vi "Teleop.vi"(0 "Call Context":T2, 5 "Match Info":T1={"Autonomous Elapsed Seconds"=0.0, "TeleOp Elapsed Seconds"=0.0, "Disabled Elapsed Seconds"=0.0, "Visited Autonomous"=FALSE, "Visited TeleOp"=FALSE, "Visited Disabled"=FALSE, "Autonomous Settings"={"Autonomous Style"=enum."Independent", "VI Refnum"=refnum}}) -> ()   [LabVIEW 2020]
doc: "This VI is called for each TeleOp packet received from the DS where the robot is not disabled. It is often used to read from the joysticks and update I/O or to update setpoints for timed control loops. It should complete and return within 20 milliseconds or it may miss DS packets."
uses:
  <vilib>/Rock Robotics/WPI/DriverStation/WPI_DriverStationDerivedRobotMode.ctl
  <vilib>/Rock Robotics/WPI/DriverStation/WPI_DriverStationMatch Info.ctl
  <vilib>/Rock Robotics/WPI/Utilities/WPI_GetSetVariantRefNum.vi
  <vilib>/Rock Robotics/Network Tables/NT Read Boolean.vi
  <vilib>/Rock Robotics/Network Tables/NT Read Number.vi
  LX.vi
panel:
  out "Sample Slider 0":dbl(slide) scale=0.0..5.0
  out "Sample Boolean 1":bool
  out "Sample Boolean 0":bool
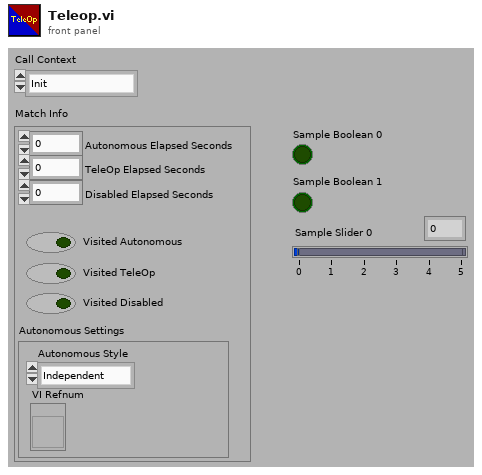
[diagram p1: front panel]
types:
  T1 = typedef "WPI_DriverStationMatch Info.ctl" = cluster{"Autonomous Elapsed Seconds":dbl, "TeleOp Elapsed Seconds":dbl, "Disabled Elapsed Seconds":dbl, "Visited Autonomous":bool, "Visited TeleOp":bool, "Visited Disabled":bool, "Autonomous Settings":cluster{"Autonomous Style":enum16{"Iterative", "Independent"}, "VI Refnum":refnum<vi>}}
  T2 = typedef "WPI_DriverStationDerivedRobotMode.ctl" = enum16{"Init", "Execute", "Stop"}
  T3 = typedef "WPI_JoystickDevRef.ctl" = cluster{"Device":T4}
  T4 = typedef "WPI_JoystickDeviceEnum.ctl" = enum16{"USB 0", "USB 1", "USB 2", "USB 3", "USB 4", "USB 5"}
  T5 = typedef "WPI_RobotDriveDevRef.ctl" = cluster{"DevStatus":errorcluster, "Motors[]":T6[], "Square Inputs":bool, "Max Output":dbl}
  T6 = typedef "WPI_MotorControlDeviceRef.ctl" = cluster{"DeviceStatus":errorcluster, "Type":T7, "PWM":cluster{"PWM Channel":T8, "DeadBand":T9}, "CAN":cluster{"Device Number":u8, "SetOutput VI Ref":variant, "GetOutput VI Ref":variant, "Enable VI Ref":variant, "Disable VI Ref":variant, "Data":variant}, "Invert":bool, "DIO PWM":cluster{"PWM \"Enable\" Channel":T8, "DIOChannel":T10, "PWM Rate":dbl}}
  T7 = typedef "WPI_MotorControlType.ctl" = enum16{"PWM", "CAN", "DIO PWM"}
  T8 = typedef "FPGA_DIOPWMChannel.ctl" = enum8{"PWM 0", "PWM 1", "PWM 2", "PWM 3", "PWM 4", "PWM 5", "PWM 6", "PWM 7", "PWM 8", "PWM 9", "PWM MXP 0", "PWM MXP 1", "PWM MXP 2", "PWM MXP 3", "PWM MXP 4", "PWM MXP 5", "PWM MXP 6", "PWM MXP 7", "PWM MXP 8", "PWM MXP 9", "Invalid"}
  T9 = typedef "WPI_PWMDeadband.ctl" = cluster{"Name":string, "maxPositivePwm":i32, "minPositivePwm":i32, "centerPwm":i32, "maxNegativePwm":i32, "minNegativePwm":i32, "angularRange":u16}
  T10 = typedef "FPGA_DIOChannel.ctl" = enum8{"DIO 0", "DIO 1", "DIO 2", "DIO 3", "DIO 4", "DIO 5", "DIO 6", "DIO 7", "DIO 8", "DIO 9", "DIO MXP 0", "DIO MXP 1", "DIO MXP 2", "DIO MXP 3", "DIO MXP 4", "DIO MXP 5", "DIO MXP 6", "DIO MXP 7", "DIO MXP 8", "DIO MXP 9", "DIO MXP 10", "DIO MXP 11", "DIO MXP 12", "DIO MXP 13", "DIO MXP 14", "DIO MXP 15", "SPI Port CS1", "SPI Port CS2", "SPI Port CS3", "SPI Port MISO", "SPI Port MOSI", "Invalid"}
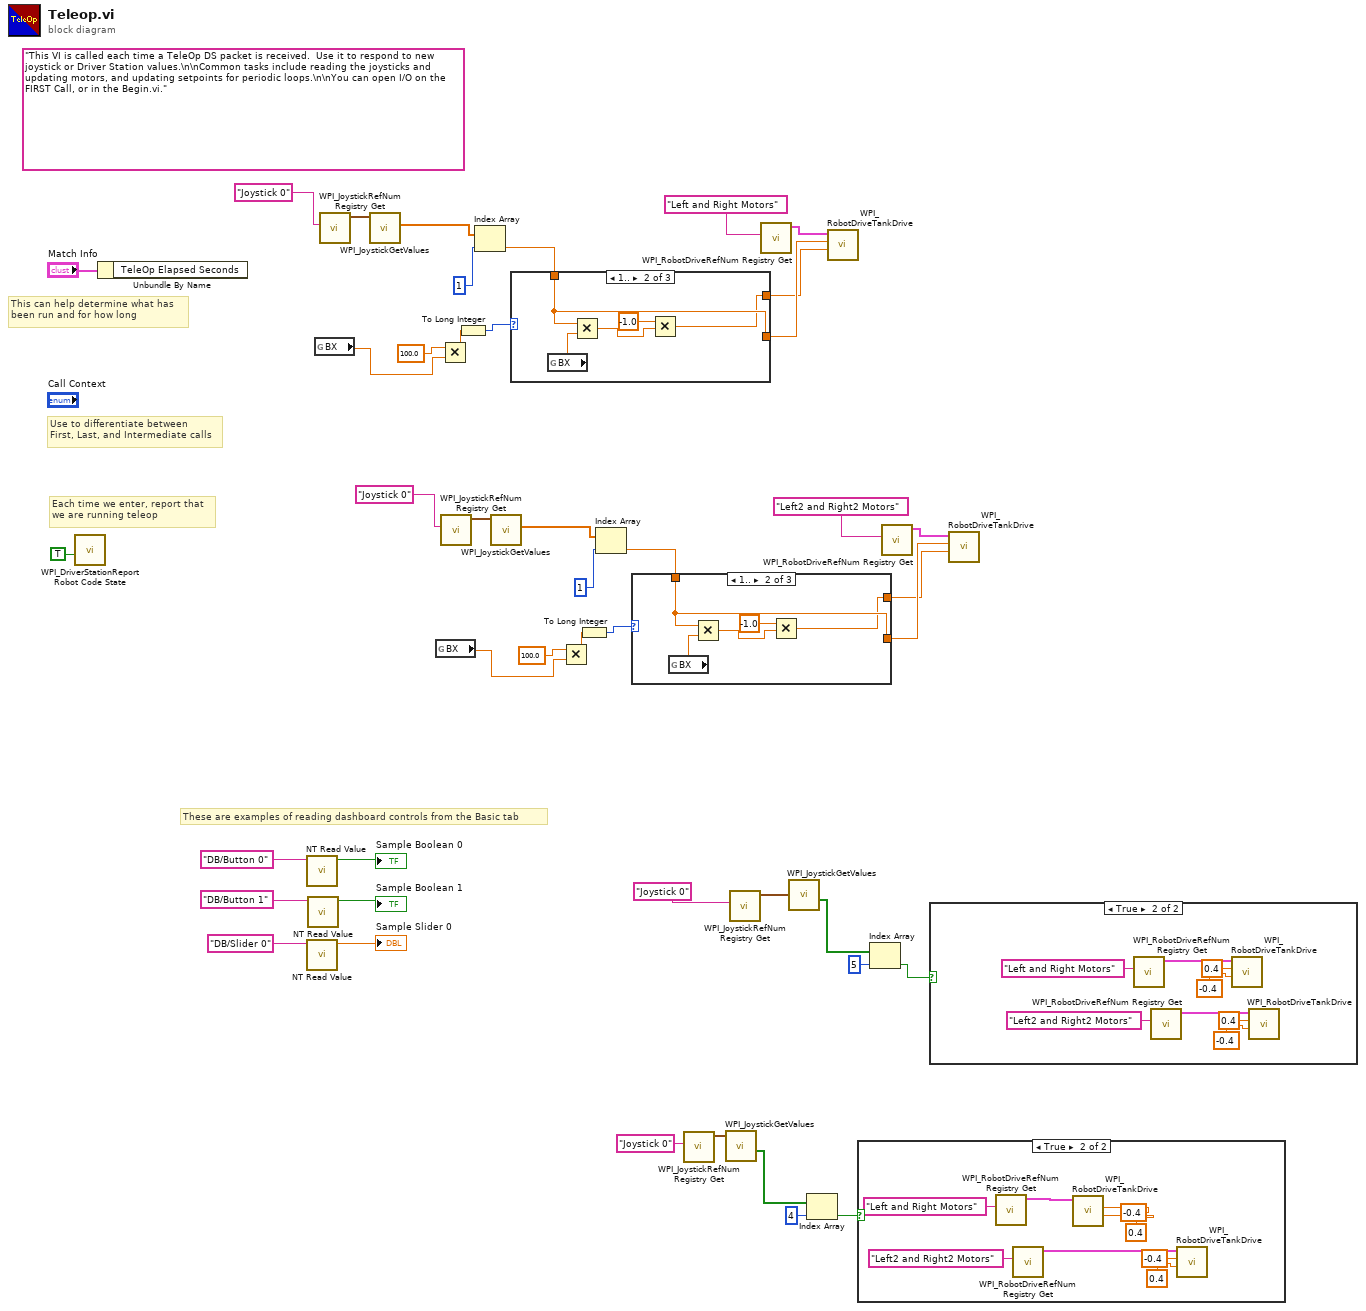
[diagram p0: block diagram]
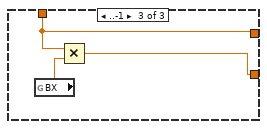
[diagram p3: hidden frame]
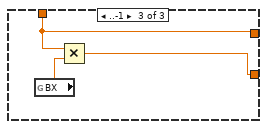
[diagram p5: hidden frame]
diagram:
  (unwired) "This VI is called each time a TeleOp DS packet is received.  Use it to respond to new joystick or Driver Station values.\n\nCommon tasks include reading the joysticks and updating motors, and updating setpoints for periodic loops.\n\nYou can open I/O on the FIRST Call, or in the Begin.vi."
  # "These are examples of reading dashboard controls from the Basic tab"
  # "Each time we enter, report that\nwe are running teleop"
  # "Use to differentiate between\nFirst, Last, and Intermediate calls"
  # "This can help determine what has\nbeen run and for how long"
  n1 = call <vilib>:"WPI_DriverStationReport Robot Code State.vi"("TeleOp"=TRUE ("Autonomous")) -> ()  [unwired: 10 in, 1 out]
  n2 = Unbundle By Name("Match Info") -> ()  [unwired: 1 out]
  n3 = call-poly <vilib>:"NT Read Value.vi"("Name"="DB/Button 0" ("refnum name")) -> ("Boolean"=→"Sample Boolean 0":bool)  [unwired: 9 in, 1 out]
  n4 = call-poly <vilib>:"NT Read Value.vi"("Name"="DB/Slider 0" ("refnum name")) -> ("Numeric"=→"Sample Slider 0":dbl)  [unwired: 9 in, 1 out]
  n5 = call-poly <vilib>:"NT Read Value.vi"("Name"="DB/Button 1" ("refnum name")) -> ("Boolean"=→"Sample Boolean 1":bool)  [unwired: 9 in, 1 out]
  n6 = global read "LX.vi" "BX"() -> (w23:dbl)
  n7 = call <vilib>:"WPI_JoystickRefNum Registry Get.vi"("refnum name"="Joystick 0") -> ("JoystickDevRef"=w17:T3)  [unwired: 1 in, 9 out]
  n8 = call <vilib>:"WPI_JoystickGetValues.vi"("JoystickDevRef"=w17) -> ("Axes"=w19:dbl[])  [unwired: 6 in, 4 out]
  n9 = global read "LX.vi" "BX"() -> (w10:dbl)
  n10 = Multiply(x=100.0, y=w23) -> (x*y=w22:dbl)
  n11 = call <vilib>:"WPI_JoystickRefNum Registry Get.vi"("refnum name"="Joystick 0") -> ("JoystickDevRef"=w4:T3)  [unwired: 1 in, 9 out]
  n12 = To Long Integer(number=w22) -> (32bit integer=w21:i32)
  n13 = Index Array(array=w19, index=1) -> (element=w16:dbl)
  n14 = call <vilib>:"WPI_JoystickGetValues.vi"("JoystickDevRef"=w4) -> ("Axes"=w6:dbl[])  [unwired: 6 in, 4 out]
  n15 = case shown="1.." w21 {
    tunnel: w16 -> [w45 w47 w51]
    tunnel: [w45 w47 w52] -> w15
    tunnel: [w45 w46 w51] -> w14
    frame 0, Default {
    }
    frame 1.. {
      n16 = global read "LX.vi" "BX"() -> (w50:dbl)
      n17 = Multiply(x=w47, y=w50) -> (x*y=w48:dbl)
      n18 = Multiply(x=-1.0, y=w48) -> (x*y=w46:dbl)
    }
    frame ..-1 {
      n19 = global read "LX.vi" "BX"() -> (w53:dbl)
      n20 = Multiply(x=w51, y=w53) -> (x*y=w52:dbl)
    }
  }
  n21 = Multiply(x=100.0, y=w10) -> (x*y=w9:dbl)
  n22 = To Long Integer(number=w9) -> (32bit integer=w8:i32)
  n23 = Index Array(array=w6, index=1) -> (element=w3:dbl)
  n24 = case shown="1.." w8 {
    tunnel: w3 -> [w54 w56 w60]
    tunnel: [w54 w56 w61] -> w2
    tunnel: [w54 w55 w60] -> w1
    frame 0, Default {
    }
    frame 1.. {
      n25 = global read "LX.vi" "BX"() -> (w59:dbl)
      n26 = Multiply(x=w56, y=w59) -> (x*y=w57:dbl)
      n27 = Multiply(x=-1.0, y=w57) -> (x*y=w55:dbl)
    }
    frame ..-1 {
      n28 = global read "LX.vi" "BX"() -> (w62:dbl)
      n29 = Multiply(x=w60, y=w62) -> (x*y=w61:dbl)
    }
  }
  n30 = call <vilib>:"WPI_JoystickRefNum Registry Get.vi"("refnum name"="Joystick 0") -> ("JoystickDevRef"=w33:T3)  [unwired: 9 in, 1 out]
  n31 = call <vilib>:"WPI_JoystickGetValues.vi"("JoystickDevRef"=w33) -> ("Buttons"=w32:bool[])  [unwired: 6 in, 4 out]
  n32 = call <vilib>:"WPI_JoystickRefNum Registry Get.vi"("refnum name"="Joystick 0") -> ("JoystickDevRef"=w29:T3)  [unwired: 9 in, 1 out]
  n33 = call <vilib>:"WPI_RobotDriveRefNum Registry Get.vi"("refnum name"="Left and Right Motors") -> ("RobotDriveDevRef"=w35:T5)  [unwired: 1 in, 9 out]
  n34 = call <vilib>:"WPI_JoystickGetValues.vi"("JoystickDevRef"=w29) -> ("Buttons"=w28:bool[])  [unwired: 6 in, 4 out]
  n35 = Index Array(array=w32, index=4) -> (element=w25:bool)
  n36 = call <vilib>:"WPI_RobotDriveTankDrive.vi"("Right axis value"=w14, "Left axis value"=w15, "RobotDriveDevRef"=w35) -> ()  [unwired: 6 in, 3 out]
  n37 = case shown="True" w25 {
    frame False {
    }
    frame True {
      n38 = call <vilib>:"WPI_RobotDriveRefNum Registry Get.vi"("refnum name"="Left and Right Motors") -> ("RobotDriveDevRef"=w70:T5)  [unwired: 9 in, 1 out]
      n39 = call <vilib>:"WPI_RobotDriveRefNum Registry Get.vi"("refnum name"="Left2 and Right2 Motors") -> ("RobotDriveDevRef"=w69:T5)  [unwired: 9 in, 1 out]
      n40 = call <vilib>:"WPI_RobotDriveTankDrive.vi"("Right axis value"=0.4, "Left axis value"=-0.4, "RobotDriveDevRef"=w70) -> ()  [unwired: 6 in, 3 out]
      n41 = call <vilib>:"WPI_RobotDriveTankDrive.vi"("Right axis value"=0.4, "Left axis value"=-0.4, "RobotDriveDevRef"=w69) -> ()  [unwired: 6 in, 3 out]
    }
  }
  n42 = Index Array(array=w28, index=5) -> (element=w26:bool)
  n43 = call <vilib>:"WPI_RobotDriveRefNum Registry Get.vi"("refnum name"="Left2 and Right2 Motors") -> ("RobotDriveDevRef"=w12:T5)  [unwired: 1 in, 9 out]
  n44 = case shown="True" w26 {
    frame False {
    }
    frame True {
      n45 = call <vilib>:"WPI_RobotDriveRefNum Registry Get.vi"("refnum name"="Left and Right Motors") -> ("RobotDriveDevRef"=w78:T5)  [unwired: 9 in, 1 out]
      n46 = call <vilib>:"WPI_RobotDriveRefNum Registry Get.vi"("refnum name"="Left2 and Right2 Motors") -> ("RobotDriveDevRef"=w77:T5)  [unwired: 9 in, 1 out]
      n47 = call <vilib>:"WPI_RobotDriveTankDrive.vi"("Right axis value"=-0.4, "Left axis value"=0.4, "RobotDriveDevRef"=w78) -> ()  [unwired: 6 in, 3 out]
      n48 = call <vilib>:"WPI_RobotDriveTankDrive.vi"("Right axis value"=-0.4, "Left axis value"=0.4, "RobotDriveDevRef"=w77) -> ()  [unwired: 6 in, 3 out]
    }
  }
  n49 = call <vilib>:"WPI_RobotDriveTankDrive.vi"("Right axis value"=w1, "Left axis value"=w2, "RobotDriveDevRef"=w12) -> ()  [unwired: 6 in, 3 out]
